vi "TCP&IP.vi"(2 "Data To TCP":string, 3 "确定按钮":bool, 4 "IP":string) -> (1 "Data From TCP":string)   [LabVIEW 2014]
panel:
  out "连接ID":refnum<k5>
  out "错误输出":errorcluster
  in  "Port":u16
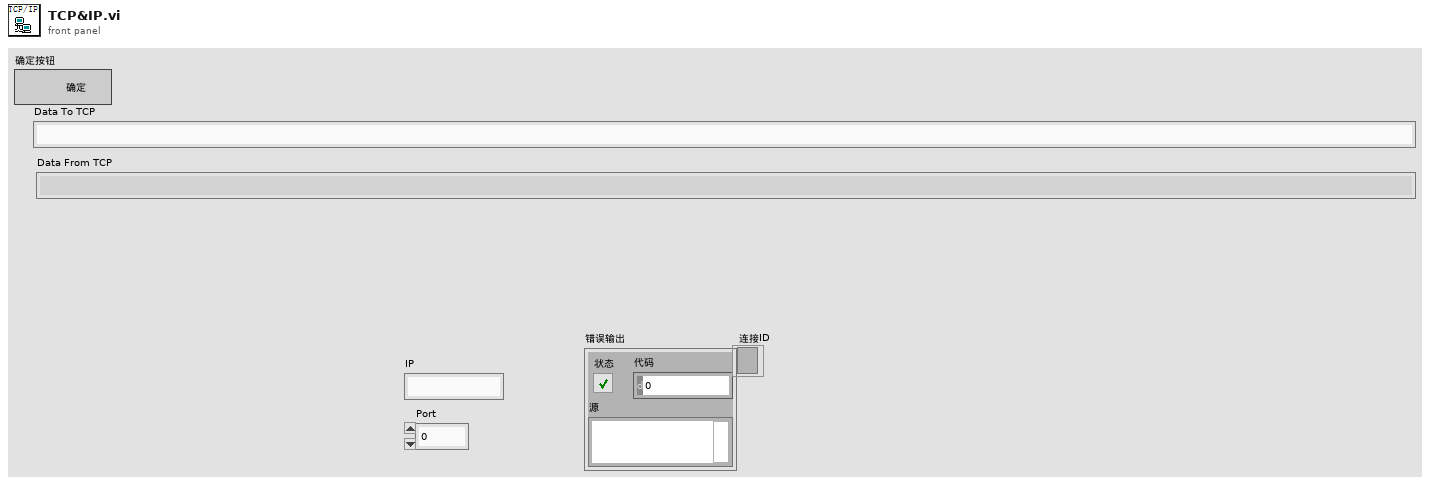
[diagram p1: front panel]
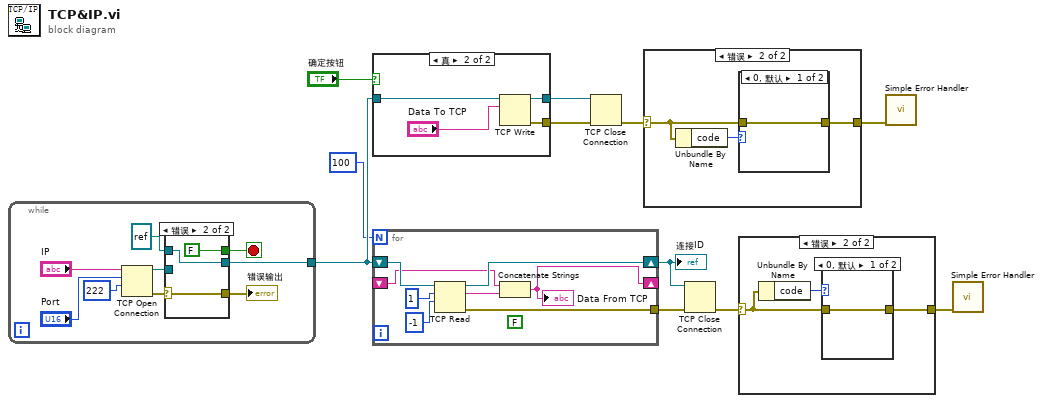
[diagram p0: block diagram]
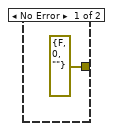
[diagram p3: hidden frame]
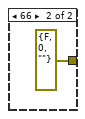
[diagram p4: hidden frame]
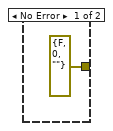
[diagram p5: hidden frame]
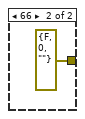
[diagram p6: hidden frame]
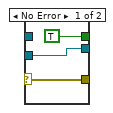
[diagram p7: hidden frame]
diagram:
  n1 = while {
    tunnel: [w14] -> w11
    stop <- w16 stop-if-true
    n2 = TCP Open Connection(address="IP", remote port or service name="Port", timeout ms (60000)=222 ("超时毫秒(60000)")) -> (connection ID=w13:refnum<k5>, error out=w17:errorcluster)  [unwired: 2 in]
    n3 = case shown="错误" w17 {
      selector: w17 -> [w22 w25]
      tunnel: [TRUE FALSE] -> w16
      tunnel: [w22 w25] -> w15
      tunnel: [w21 w24] -> w14
      tunnel: w13 -> [w21 _]
      tunnel: refnum<k5> refnum ("连接ID") -> [_ w24]
      frame No Error {
      }
      frame Error {
      }
    }
    "错误输出" <- w15
  }
  n4 = case shown="真" "确定按钮" {
    tunnel: w11 -> [_ w30]
    tunnel: [_ w28] -> w10
    tunnel: [_ w27] -> w9
    frame False {
    }
    frame True {
      n5 = TCP Write(connection ID=w30, data in="Data To TCP") -> (connection ID out=w28:refnum<k5>, error out=w27:errorcluster)  [unwired: 2 in, 1 out]
    }
  }
  n6 = for {
    N: 100 -> [_]
    shift-right: [w35] -> w8
    shift-left: w11 -> [w38]
    shift-right: [w33] -> _
    shift-left: _ -> [w32]
    tunnel: [w31] -> w7
    (unwired) FALSE
    n7 = TCP Read(connection ID=w38, bytes to read=1 ("读取的字节"), 9:-1 ("超时毫秒(25000)")) -> (connection ID out=w35:refnum<k5>, data out=w34:string, error out=w31:errorcluster)  [unwired: 2 in]
    n8 = Concatenate Strings(w32, w34) -> (w33:string)
    "Data From TCP" <- w33
  }
  "连接ID" <- w8
  n9 = TCP Close Connection(connection ID=w10, error in (no error)=w9) -> (error out=w3:errorcluster)  [unwired: 1 in, 1 out]
  n10 = case shown="错误" w3 {
    selector: w3 -> [_ w40]
    tunnel: [errorcluster {"status"=FALSE, "code"=0, "source"=""} ("错误常量") w41] -> w4
    frame No Error {
    }
    frame Error {
      n11 = Unbundle By Name(w40) -> ("code"=w42:i32)
      n12 = case shown="0, 默认" w42 {
        tunnel: [w43 errorcluster {"status"=FALSE, "code"=0, "source"=""} ("错误常量")] -> w41
        tunnel: w40 -> [w43 _]
        frame 0, Default {
        }
        frame 66 {
        }
      }
    }
  }
  n13 = TCP Close Connection(connection ID=w8, error in (no error)=w7) -> (error out=w6:errorcluster)  [unwired: 1 in, 1 out]
  n14 = case shown="错误" w6 {
    selector: w6 -> [_ w46]
    tunnel: [errorcluster {"status"=FALSE, "code"=0, "source"=""} ("错误常量") w47] -> w5
    frame No Error {
    }
    frame Error {
      n15 = Unbundle By Name(w46) -> ("code"=w48:i32)
      n16 = case shown="0, 默认" w48 {
        tunnel: [w49 errorcluster {"status"=FALSE, "code"=0, "source"=""} ("错误常量")] -> w47
        tunnel: w46 -> [w49 _]
        frame 0, Default {
        }
        frame 66 {
        }
      }
    }
  }
  n17 = call <vilib>:"Simple Error Handler.vi"("error in (no error)"=w4) -> ()  [unwired: 4 in, 5 out]
  n18 = call <vilib>:"Simple Error Handler.vi"("error in (no error)"=w5) -> ()  [unwired: 4 in, 5 out]
